vi "Filter Wheel Position Test.vi"(8 "error in (no error)":errorcluster, 10 "Position":u8, 11 "Session Handle in":T1) -> (0 "error out":errorcluster, 2 "Passed?":bool, 3 "Session Handle out":T1 caption="Gas")   [LabVIEW 2015, in "PAS.lvclass"]
uses:
  PAS.lvclass
  Typedefs/Session Handle.ctl
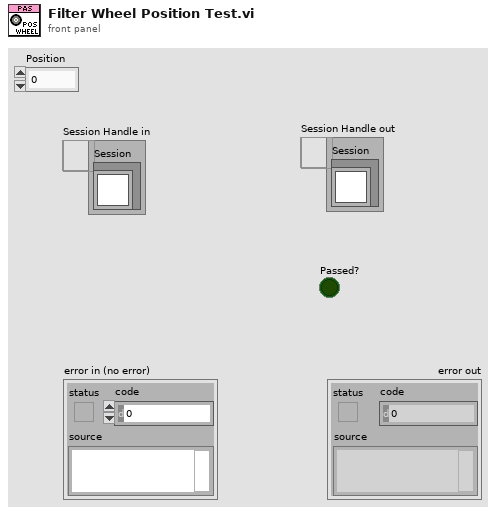
[diagram p1: front panel]
types:
  T1 = typedef "PAS.lvclass/Session Handle.ctl" = refnum<data-value>
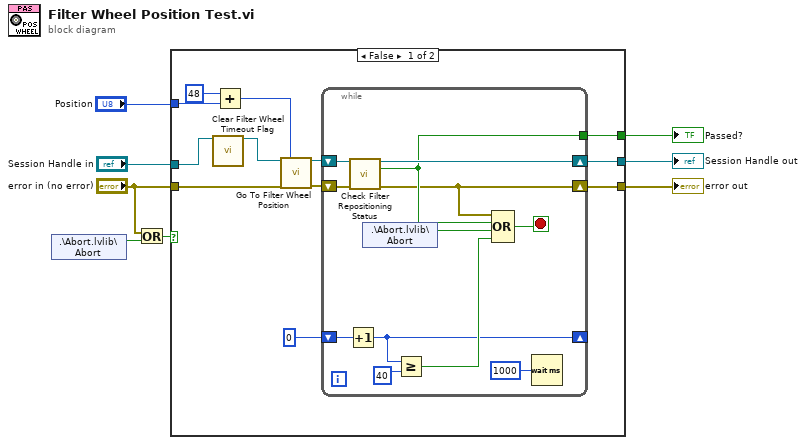
[diagram p0: block diagram]
diagram:
  n1 = shared-variable ".\\Abort.lvlib\\Abort"() -> (w2:bool)  [unwired: 1 in, 1 out]
  n2 = Or(x="error in (no error)", y=w2) -> (x .or. y?=w4:bool)
  n3 = case shown="False" w4 {
    tunnel: [w20 w33] -> w8
    tunnel: [w19 _] -> w7
    tunnel: [w17 w34] -> w6
    tunnel: "Session Handle in" -> [w16 w34]
    tunnel: "error in (no error)" -> [w12 w33]
    tunnel: "Position" -> [w11 _]
    frame False {
      n4 = call "Clear Filter Wheel Timeout Flag.vi"("Session Handle in"=w16) -> ("Session Handle out"=w15:T1)  [unwired: 11 in, 3 out]
      n5 = Add(x=u8 48, y=w11) -> (x+y=w9:u8)
      n6 = call "Go To Filter Wheel Position.vi"("Session Handle in"=w15, "Positions"=w9, "error in (no error)"=w12) -> ("Session Handle out"=w14:T1, "error out"=w13:errorcluster)  [unwired: 10 in, 1 out]
      n7 = while {
        shift-right: [w22] -> w20
        shift-left: w13 -> [w26]
        shift-right: [w24] -> w17
        shift-left: w14 -> [w25]
        tunnel: [w23] -> w19
        shift-right: [w27] -> _
        shift-left: u32 0 ("milliseconds to wait") -> [w30]
        stop <- w31 stop-if-true
        n8 = Increment(x=w30) -> (x+1=w27:u32)
        n9 = call "Check Filter Repositioning Status.vi"("Session Handle in"=w25, "error in (no error)"=w26) -> ("Session Handle out"=w24:T1, "Success?"=w23:bool, "error out"=w22:errorcluster)  [unwired: 11 in]
        n10 = shared-variable ".\\Abort.lvlib\\Abort"() -> (w21:bool)  [unwired: 1 in, 1 out]
        n11 = Greater Or Equal?(x=w27, y=u32 40) -> (x >= y?=w28:bool)
        n12 = Compound Arithmetic op=OR(w22, w23, w21, w28) -> (w31:bool)
        n13 = Wait (ms)(milliseconds to wait=u32 1000) -> ()  [unwired: 1 out]
      }
    }
    frame True {
    }
  }
  "error out" <- w8
  "Passed?" <- w7
  "Session Handle out" <- w6
